vi "Other side RTS CTS Exchange.vi"() -> ()   [LabVIEW 2012]
uses:
  <instrlib>/niUSRP/niUSRP Fetch Rx Data (CDB).vi
  <vilib>/Analysis/2dsp.llb/Complex FFT.vi
  <vilib>/addons/Modulation/Digital/General/MT Map QAM Symbols to Bits.vi
  <vilib>/addons/Modulation/Digital/General/MT Map Bits to QAM Symbols.vi
  <instrlib>/niUSRP/niUSRP Write Tx Data (CDB).vi
  <vilib>/Analysis/2dsp.llb/Inverse Complex FFT.vi
  <vilib>/Waveform/DWDTOps.llb/DWDT Binary U8 to Digital.vi
  <vilib>/Waveform/DWDTOps.llb/DWDT Digital to Analog.vi
  <vilib>/Analysis/NI_AALPro.lvlib
  <vilib>/addons/Modulation/niDMT.lvlib
panel:
  out "Received Signal":waveform(dbl)(graph)
  out "analog waveform":waveform(dbl)
  out "CTS is send":bool
  out "sum":i8
  out "output array 2":i8[](array[numeric])
  out "output array 3":i8[](array[numeric])
  in  "stop":bool
  out "Reference Signal \n(RTS) Received":bool
  in  "Tab Control":enum32{"Parameters", "Debug", "CFO"}(tab)
  in  "Device names":refnum<k15>="192.168.10.3"
  in  "Active antenna":string="RX1"
  in  "Gain":dbl=3.0 format="%#_6f"
  in  "Carrier frequency":dbl=910000000.0 format="%#_6p"
  in  "IQ rate":dbl=5000000.0 format="%#_6p"
  in  "Number of samples":i64=1600
  out "Coerced IQ rate":dbl=100000.0 format="%#_6p"
  out "error out":errorcluster
  out "error out 2":errorcluster
  out "CFOest (Hz)":dbl[](array[numeric])
  out "Magnitude":dbl[](graph)
  out "Phase":dbl[](graph)
  out "FFT {X}":dbl[](graph)
  out "theta":dbl[](graph)
  out "Unequalized Data":cdb[](graph)
  out "Equalized Data":cdb[](graph)
  out "output bit stream":i8[][](array[numeric])
  out "Received Message":string
  out "millisecond timer to \n    Receive Signal":u32
  in  "Tab Control 2":enum32{"Parameters", "Debug"}(tab)
  out "coerced IQ rate":dbl=100000.0 format="%#_6p"
  in  "error in (no error)":errorcluster
  out "error out 3":errorcluster
  out "X":cdb[](array[numeric])
  out "Array out":cdb[](array[numeric])
  out "Interleaved Output":cdb[](array[numeric])
  out "Output with CP":cdb[](array[numeric])
  out "Data Size":i32
  out "Reference Symbols \n         Added":i32
  out "After Zero \n  Padding":i32
  out "After CP":i32
  out "Outgoing Constellation":cdb[](graph)=[-0.7071067811865476-0.7071067811865476i, -0.7071067811865476-0.7071067811865476i, -0.7071067811865476-0.7071067811865476i, 0.7071067811865476-0.7071067811865476i, 0.7071067811865476-0.7071067811865476i, 0.7071067811865476+0.7071067811865476i, 0.7071067811865476-0.7071067811865476i, -0.7071067811865476-0.7071067811865476i, 0.7071067811865476+0.7071067811865476i, -0.7071067811865476+0.7071067811865476i, -0.7071067811865476-0.7071067811865476i, -0.7071067811865476+0.7071067811865476i, -0.7071067811865476+0.7071067811865476i, 0.7071067811865476-0.7071067811865476i, -0.7071067811865476+0.7071067811865476i, -0.7071067811865476+0.7071067811865476i, 0.7071067811865476-0.7071067811865476i, -0.7071067811865476+0.7071067811865476i, -0.7071067811865476-0.7071067811865476i, 0.7071067811865476-0.7071067811865476i, 0.7071067811865476+0.7071067811865476i, -0.7071067811865476-0.7071067811865476i, -0.7071067811865476-0.7071067811865476i, 0.7071067811865476-0.7071067811865476i, -0.7071067811865476-0.7071067811865476i, 0.7071067811865476-0.7071067811865476i, 0.7071067811865476-0.7071067811865476i, 0.7071067811865476+0.7071067811865476i, 0.7071067811865476+0.7071067811865476i, -0.7071067811865476-0.7071067811865476i, -0.7071067811865476+0.7071067811865476i, -0.7071067811865476+0.7071067811865476i, 0.7071067811865476-0.7071067811865476i, -0.7071067811865476-0.7071067811865476i, -0.7071067811865476+0.7071067811865476i, -0.7071067811865476-0.7071067811865476i, -0.7071067811865476+0.7071067811865476i, 0.7071067811865476-0.7071067811865476i, 0.7071067811865476+0.7071067811865476i, 0.7071067811865476+0.7071067811865476i, 0.7071067811865476-0.7071067811865476i, -0.7071067811865476-0.7071067811865476i, -0.7071067811865476+0.7071067811865476i, -0.7071067811865476+0.7071067811865476i, -0.7071067811865476-0.7071067811865476i, -0.7071067811865476-0.7071067811865476i, -0.7071067811865476+0.7071067811865476i, -0.7071067811865476+0.7071067811865476i, -0.7071067811865476+0.7071067811865476i, -0.7071067811865476+0.7071067811865476i, 0.7071067811865476+0.7071067811865476i, 0.7071067811865476+0.7071067811865476i, 0.7071067811865476+0.7071067811865476i, 0.7071067811865476-0.7071067811865476i, 0.7071067811865476-0.7071067811865476i, -0.7071067811865476+0.7071067811865476i, -0.7071067811865476+0.7071067811865476i, -0.7071067811865476+0.7071067811865476i, -0.7071067811865476-0.7071067811865476i, 0.7071067811865476-0.7071067811865476i, -0.7071067811865476+0.7071067811865476i, -0.7071067811865476+0.7071067811865476i, -0.7071067811865476-0.7071067811865476i, -0.7071067811865476+0.7071067811865476i, -0.7071067811865476-0.7071067811865476i, 0.7071067811865476+0.7071067811865476i, 0.7071067811865476+0.7071067811865476i, 0.7071067811865476+0.7071067811865476i, -0.7071067811865476-0.7071067811865476i, 0.7071067811865476-0.7071067811865476i, -0.7071067811865476+0.7071067811865476i, -0.7071067811865476-0.7071067811865476i, -0.7071067811865476+0.7071067811865476i, 0.7071067811865476+0.7071067811865476i, 0.7071067811865476-0.7071067811865476i, -0.7071067811865476+0.7071067811865476i, -0.7071067811865476-0.7071067811865476i, 0.7071067811865476-0.7071067811865476i, 0.7071067811865476-0.7071067811865476i, -0.7071067811865476-0.7071067811865476i, 0.7071067811865476-0.7071067811865476i, 0.7071067811865476-0.7071067811865476i, 0.7071067811865476-0.7071067811865476i, 0.7071067811865476+0.7071067811865476i, 0.7071067811865476-0.7071067811865476i, -0.7071067811865476+0.7071067811865476i, 0.7071067811865476+0.7071067811865476i, 0.7071067811865476+0.7071067811865476i, -0.7071067811865476-0.7071067811865476i, 0.7071067811865476+0.7071067811865476i, -0.7071067811865476-0.7071067811865476i, 0.7071067811865476-0.7071067811865476i, 0.7071067811865476+0.7071067811865476i, -0.7071067811865476+0.7071067811865476i, -0.7071067811865476+0.7071067811865476i, -0.7071067811865476-0.7071067811865476i, 0.7071067811865476-0.7071067811865476i, -0.7071067811865476-0.7071067811865476i, -0.7071067811865476+0.7071067811865476i, 0.7071067811865476-0.7071067811865476i, -0.7071067811865476+0.7071067811865476i, 0.7071067811865476-0.7071067811865476i, 0.7071067811865476-0.7071067811865476i, 0.7071067811865476+0.7071067811865476i, -0.7071067811865476+0.7071067811865476i, -0.7071067811865476-0.7071067811865476i, -0.7071067811865476+0.7071067811865476i, -0.7071067811865476-0.7071067811865476i, 0.7071067811865476-0.7071067811865476i, 0.7071067811865476+0.7071067811865476i, -0.7071067811865476+0.7071067811865476i, -0.7071067811865476-0.7071067811865476i, -0.7071067811865476-0.7071067811865476i, -0.7071067811865476-0.7071067811865476i, -0.7071067811865476-0.7071067811865476i, 0.7071067811865476+0.7071067811865476i, 0.7071067811865476+0.7071067811865476i, -0.7071067811865476+0.7071067811865476i, -0.7071067811865476-0.7071067811865476i, 0.7071067811865476-0.7071067811865476i, -0.7071067811865476-0.7071067811865476i, -0.7071067811865476-0.7071067811865476i, 0.7071067811865476-0.7071067811865476i, 0.7071067811865476+0.7071067811865476i, 0.7071067811865476-0.7071067811865476i, -0.7071067811865476-0.7071067811865476i, 0.7071067811865476-0.7071067811865476i, -0.7071067811865476+0.7071067811865476i, 0.7071067811865476-0.7071067811865476i, -0.7071067811865476+0.7071067811865476i, 0.7071067811865476+0.7071067811865476i, 0.7071067811865476+0.7071067811865476i, -0.7071067811865476+0.7071067811865476i, 0.7071067811865476+0.7071067811865476i, 0.7071067811865476-0.7071067811865476i, 0.7071067811865476-0.7071067811865476i, -0.7071067811865476+0.7071067811865476i, -0.7071067811865476-0.7071067811865476i, -0.7071067811865476+0.7071067811865476i, 0.7071067811865476-0.7071067811865476i, 0.7071067811865476-0.7071067811865476i, 0.7071067811865476+0.7071067811865476i, -0.7071067811865476-0.7071067811865476i, -0.7071067811865476-0.7071067811865476i, 0.7071067811865476+0.7071067811865476i, -0.7071067811865476-0.7071067811865476i, -0.7071067811865476-0.7071067811865476i, 0.7071067811865476-0.7071067811865476i, -0.7071067811865476+0.7071067811865476i, 0.7071067811865476-0.7071067811865476i, -0.7071067811865476-0.7071067811865476i, 0.7071067811865476+0.7071067811865476i, -0.7071067811865476+0.7071067811865476i, -0.7071067811865476+0.7071067811865476i, -0.7071067811865476+0.7071067811865476i, 0.7071067811865476+0.7071067811865476i, 0.7071067811865476-0.7071067811865476i, 0.7071067811865476+0.7071067811865476i, -0.7071067811865476-0.7071067811865476i, 0.7071067811865476-0.7071067811865476i, 0.7071067811865476+0.7071067811865476i, -0.7071067811865476-0.7071067811865476i, -0.7071067811865476+0.7071067811865476i, 0.7071067811865476-0.7071067811865476i, 0.7071067811865476-0.7071067811865476i, 0.7071067811865476-0.7071067811865476i, -0.7071067811865476-0.7071067811865476i, 0.7071067811865476-0.7071067811865476i, 0.7071067811865476+0.7071067811865476i, 0.7071067811865476-0.7071067811865476i, -0.7071067811865476+0.7071067811865476i, 0.7071067811865476-0.7071067811865476i, 0.7071067811865476+0.7071067811865476i, 0.7071067811865476-0.7071067811865476i, 0.7071067811865476+0.7071067811865476i, 0.7071067811865476-0.7071067811865476i, 0.7071067811865476+0.7071067811865476i, 0.7071067811865476+0.7071067811865476i, 0.7071067811865476+0.7071067811865476i, -0.7071067811865476+0.7071067811865476i, 0.7071067811865476+0.7071067811865476i, 0.7071067811865476+0.7071067811865476i, 0.7071067811865476-0.7071067811865476i, 0.7071067811865476+0.7071067811865476i, -0.7071067811865476-0.7071067811865476i, 0.7071067811865476+0.7071067811865476i, 0.7071067811865476+0.7071067811865476i, 0.7071067811865476-0.7071067811865476i, -0.7071067811865476+0.7071067811865476i, -0.7071067811865476-0.7071067811865476i, 0.7071067811865476+0.7071067811865476i, 0.7071067811865476-0.7071067811865476i, 0.7071067811865476-0.7071067811865476i, 0.7071067811865476-0.7071067811865476i, -0.7071067811865476-0.7071067811865476i, 0.7071067811865476+0.7071067811865476i, 0.7071067811865476+0.7071067811865476i, -0.7071067811865476-0.7071067811865476i, -0.7071067811865476+0.7071067811865476i, -0.7071067811865476-0.7071067811865476i, 0.7071067811865476-0.7071067811865476i, 0.7071067811865476-0.7071067811865476i, -0.7071067811865476+0.7071067811865476i, 0.7071067811865476-0.7071067811865476i, -0.7071067811865476-0.7071067811865476i, 0.7071067811865476-0.7071067811865476i, -0.7071067811865476+0.7071067811865476i, 0.7071067811865476+0.7071067811865476i, -0.7071067811865476+0.7071067811865476i, -0.7071067811865476+0.7071067811865476i, 0.7071067811865476+0.7071067811865476i, 0.7071067811865476+0.7071067811865476i, 0.7071067811865476-0.7071067811865476i, 0.7071067811865476-0.7071067811865476i, -0.7071067811865476-0.7071067811865476i, -0.7071067811865476+0.7071067811865476i, 0.7071067811865476+0.7071067811865476i, -0.7071067811865476-0.7071067811865476i, -0.7071067811865476-0.7071067811865476i, -0.7071067811865476-0.7071067811865476i, -0.7071067811865476+0.7071067811865476i, 0.7071067811865476-0.7071067811865476i, -0.7071067811865476+0.7071067811865476i, 0.7071067811865476+0.7071067811865476i, 0.7071067811865476-0.7071067811865476i, -0.7071067811865476+0.7071067811865476i, -0.7071067811865476+0.7071067811865476i, 0.7071067811865476-0.7071067811865476i, -0.7071067811865476-0.7071067811865476i, -0.7071067811865476-0.7071067811865476i, -0.7071067811865476-0.7071067811865476i, 0.7071067811865476+0.7071067811865476i, 0.7071067811865476-0.7071067811865476i, -0.7071067811865476+0.7071067811865476i, 0.7071067811865476-0.7071067811865476i, 0.7071067811865476-0.7071067811865476i, 0.7071067811865476-0.7071067811865476i, -0.7071067811865476+0.7071067811865476i, 0.7071067811865476-0.7071067811865476i, -0.7071067811865476+0.7071067811865476i, 0.7071067811865476-0.7071067811865476i, 0.7071067811865476+0.7071067811865476i, 0.7071067811865476+0.7071067811865476i, 0.7071067811865476+0.7071067811865476i, -0.7071067811865476-0.7071067811865476i, 0.7071067811865476+0.7071067811865476i, -0.7071067811865476+0.7071067811865476i, 0.7071067811865476-0.7071067811865476i, -0.7071067811865476+0.7071067811865476i, -0.7071067811865476+0.7071067811865476i, 0.7071067811865476+0.7071067811865476i, -0.7071067811865476+0.7071067811865476i, 0.7071067811865476-0.7071067811865476i, 0.7071067811865476-0.7071067811865476i, -0.7071067811865476+0.7071067811865476i, -0.7071067811865476+0.7071067811865476i, -0.7071067811865476-0.7071067811865476i, -0.7071067811865476-0.7071067811865476i, -0.7071067811865476-0.7071067811865476i, -0.7071067811865476+0.7071067811865476i, 0.7071067811865476+0.7071067811865476i, -0.7071067811865476+0.7071067811865476i, -0.7071067811865476+0.7071067811865476i, 0.7071067811865476-0.7071067811865476i, 0.7071067811865476+0.7071067811865476i, -0.7071067811865476-0.7071067811865476i, 0.7071067811865476-0.7071067811865476i, 0.7071067811865476-0.7071067811865476i, -0.7071067811865476-0.7071067811865476i, 0.7071067811865476+0.7071067811865476i, 0.7071067811865476-0.7071067811865476i, -0.7071067811865476-0.7071067811865476i, 0.7071067811865476+0.7071067811865476i, -0.7071067811865476-0.7071067811865476i, -0.7071067811865476-0.7071067811865476i, 0.7071067811865476+0.7071067811865476i, -0.7071067811865476+0.7071067811865476i, -0.7071067811865476-0.7071067811865476i, -0.7071067811865476-0.7071067811865476i, -0.7071067811865476+0.7071067811865476i, -0.7071067811865476-0.7071067811865476i, -0.7071067811865476+0.7071067811865476i, 0.7071067811865476+0.7071067811865476i, 0.7071067811865476+0.7071067811865476i, -0.7071067811865476+0.7071067811865476i, 0.7071067811865476-0.7071067811865476i, 0.7071067811865476-0.7071067811865476i, -0.7071067811865476-0.7071067811865476i, -0.7071067811865476+0.7071067811865476i, 0.7071067811865476-0.7071067811865476i, -0.7071067811865476-0.7071067811865476i, 0.7071067811865476-0.7071067811865476i, -0.7071067811865476-0.7071067811865476i, 0.7071067811865476+0.7071067811865476i, 0.7071067811865476+0.7071067811865476i, -0.7071067811865476+0.7071067811865476i, -0.7071067811865476+0.7071067811865476i, 0.7071067811865476-0.7071067811865476i, 0.7071067811865476-0.7071067811865476i, -0.7071067811865476-0.7071067811865476i, -0.7071067811865476-0.7071067811865476i, 0.7071067811865476-0.7071067811865476i, 0.7071067811865476-0.7071067811865476i, 0.7071067811865476-0.7071067811865476i, 0.7071067811865476-0.7071067811865476i, 0.7071067811865476-0.7071067811865476i, 0.7071067811865476+0.7071067811865476i, 0.7071067811865476+0.7071067811865476i, -0.7071067811865476+0.7071067811865476i, -0.7071067811865476+0.7071067811865476i, 0.7071067811865476+0.7071067811865476i, 0.7071067811865476-0.7071067811865476i, 0.7071067811865476-0.7071067811865476i, -0.7071067811865476-0.7071067811865476i, -0.7071067811865476-0.7071067811865476i, 0.7071067811865476+0.7071067811865476i, 0.7071067811865476-0.7071067811865476i, -0.7071067811865476-0.7071067811865476i, 0.7071067811865476-0.7071067811865476i, -0.7071067811865476-0.7071067811865476i, 0.7071067811865476-0.7071067811865476i, 0.7071067811865476+0.7071067811865476i, 0.7071067811865476+0.7071067811865476i, -0.7071067811865476+0.7071067811865476i, -0.7071067811865476-0.7071067811865476i, 0.7071067811865476+0.7071067811865476i, -0.7071067811865476-0.7071067811865476i, 0.7071067811865476-0.7071067811865476i, 0.7071067811865476-0.7071067811865476i, -0.7071067811865476+0.7071067811865476i, 0.7071067811865476+0.7071067811865476i, -0.7071067811865476-0.7071067811865476i, -0.7071067811865476-0.7071067811865476i, -0.7071067811865476+0.7071067811865476i, -0.7071067811865476+0.7071067811865476i, -0.7071067811865476-0.7071067811865476i, -0.7071067811865476+0.7071067811865476i, -0.7071067811865476+0.7071067811865476i, 0.7071067811865476+0.7071067811865476i, -0.7071067811865476+0.7071067811865476i, 0.7071067811865476+0.7071067811865476i, 0.7071067811865476-0.7071067811865476i, 0.7071067811865476+0.7071067811865476i, -0.7071067811865476+0.7071067811865476i, 0.7071067811865476-0.7071067811865476i, -0.7071067811865476+0.7071067811865476i, -0.7071067811865476-0.7071067811865476i, 0.7071067811865476+0.7071067811865476i, 0.7071067811865476+0.7071067811865476i, 0.7071067811865476-0.7071067811865476i, -0.7071067811865476-0.7071067811865476i, -0.7071067811865476-0.7071067811865476i, -0.7071067811865476+0.7071067811865476i, 0.7071067811865476-0.7071067811865476i, -0.7071067811865476-0.7071067811865476i, 0.7071067811865476+0.7071067811865476i, -0.7071067811865476-0.7071067811865476i, -0.7071067811865476+0.7071067811865476i, 0.7071067811865476+0.7071067811865476i, 0.7071067811865476+0.7071067811865476i, -0.7071067811865476-0.7071067811865476i, 0.7071067811865476-0.7071067811865476i, -0.7071067811865476-0.7071067811865476i, -0.7071067811865476-0.7071067811865476i, 0.7071067811865476+0.7071067811865476i, 0.7071067811865476+0.7071067811865476i, -0.7071067811865476-0.7071067811865476i, -0.7071067811865476-0.7071067811865476i, -0.7071067811865476-0.7071067811865476i, -0.7071067811865476-0.7071067811865476i, 0.7071067811865476-0.7071067811865476i, 0.7071067811865476+0.7071067811865476i, 0.7071067811865476+0.7071067811865476i, -0.7071067811865476-0.7071067811865476i, -0.7071067811865476-0.7071067811865476i, -0.7071067811865476+0.7071067811865476i, -0.7071067811865476-0.7071067811865476i, -0.7071067811865476-0.7071067811865476i, 0.7071067811865476+0.7071067811865476i, -0.7071067811865476+0.7071067811865476i, -0.7071067811865476+0.7071067811865476i, -0.7071067811865476-0.7071067811865476i, 0.7071067811865476+0.7071067811865476i, -0.7071067811865476-0.7071067811865476i, 0.7071067811865476+0.7071067811865476i, 0.7071067811865476-0.7071067811865476i, 0.7071067811865476+0.7071067811865476i, 0.7071067811865476+0.7071067811865476i, 0.7071067811865476-0.7071067811865476i, -0.7071067811865476+0.7071067811865476i, -0.7071067811865476+0.7071067811865476i, 0.7071067811865476+0.7071067811865476i, -0.7071067811865476-0.7071067811865476i, 0.7071067811865476-0.7071067811865476i, -0.7071067811865476-0.7071067811865476i, -0.7071067811865476+0.7071067811865476i, 0.7071067811865476+0.7071067811865476i, -0.7071067811865476+0.7071067811865476i, -0.7071067811865476-0.7071067811865476i, 0.7071067811865476-0.7071067811865476i, -0.7071067811865476+0.7071067811865476i, -0.7071067811865476-0.7071067811865476i, -0.7071067811865476-0.7071067811865476i, 0.7071067811865476+0.7071067811865476i, -0.7071067811865476-0.7071067811865476i, -0.7071067811865476+0.7071067811865476i, 0.7071067811865476-0.7071067811865476i, 0.7071067811865476+0.7071067811865476i, 0.7071067811865476-0.7071067811865476i, 0.7071067811865476-0.7071067811865476i, 0.7071067811865476-0.7071067811865476i, -0.7071067811865476+0.7071067811865476i, 0.7071067811865476+0.7071067811865476i, -0.7071067811865476+0.7071067811865476i, -0.7071067811865476-0.7071067811865476i, 0.7071067811865476+0.7071067811865476i, -0.7071067811865476+0.7071067811865476i, 0.7071067811865476-0.7071067811865476i, -0.7071067811865476-0.7071067811865476i, -0.7071067811865476+0.7071067811865476i, -0.7071067811865476+0.7071067811865476i, -0.7071067811865476+0.7071067811865476i, -0.7071067811865476-0.7071067811865476i, 0.7071067811865476+0.7071067811865476i, -0.7071067811865476+0.7071067811865476i, 0.7071067811865476+0.7071067811865476i, -0.7071067811865476-0.7071067811865476i, 0.7071067811865476+0.7071067811865476i, -0.7071067811865476+0.7071067811865476i, 0.7071067811865476+0.7071067811865476i, -0.7071067811865476+0.7071067811865476i, 0.7071067811865476+0.7071067811865476i, 0.7071067811865476+0.7071067811865476i, 0.7071067811865476+0.7071067811865476i, 0.7071067811865476+0.7071067811865476i, 0.7071067811865476-0.7071067811865476i, 0.7071067811865476+0.7071067811865476i, -0.7071067811865476+0.7071067811865476i, 0.7071067811865476+0.7071067811865476i, -0.7071067811865476+0.7071067811865476i, 0.7071067811865476-0.7071067811865476i, 0.7071067811865476+0.7071067811865476i, -0.7071067811865476+0.7071067811865476i, 0.7071067811865476+0.7071067811865476i, -0.7071067811865476-0.7071067811865476i, 0.7071067811865476-0.7071067811865476i, -0.7071067811865476+0.7071067811865476i, -0.7071067811865476+0.7071067811865476i, -0.7071067811865476+0.7071067811865476i, -0.7071067811865476+0.7071067811865476i, 0.7071067811865476-0.7071067811865476i, 0.7071067811865476+0.7071067811865476i, -0.7071067811865476+0.7071067811865476i, 0.7071067811865476-0.7071067811865476i, -0.7071067811865476-0.7071067811865476i, -0.7071067811865476-0.7071067811865476i, -0.7071067811865476+0.7071067811865476i, 0.7071067811865476+0.7071067811865476i, -0.7071067811865476-0.7071067811865476i, -0.7071067811865476+0.7071067811865476i, -0.7071067811865476-0.7071067811865476i, 0.7071067811865476+0.7071067811865476i, 0.7071067811865476-0.7071067811865476i, 0.7071067811865476+0.7071067811865476i, 0.7071067811865476-0.7071067811865476i, 0.7071067811865476-0.7071067811865476i, 0.7071067811865476+0.7071067811865476i, -0.7071067811865476+0.7071067811865476i, -0.7071067811865476+0.7071067811865476i, -0.7071067811865476+0.7071067811865476i, 0.7071067811865476-0.7071067811865476i, 0.7071067811865476-0.7071067811865476i, -0.7071067811865476+0.7071067811865476i, -0.7071067811865476-0.7071067811865476i, -0.7071067811865476-0.7071067811865476i, 0.7071067811865476-0.7071067811865476i, -0.7071067811865476-0.7071067811865476i, 0.7071067811865476+0.7071067811865476i, 0.7071067811865476-0.7071067811865476i, -0.7071067811865476+0.7071067811865476i, 0.7071067811865476+0.7071067811865476i, 0.7071067811865476-0.7071067811865476i, -0.7071067811865476-0.7071067811865476i, -0.7071067811865476+0.7071067811865476i, -0.7071067811865476-0.7071067811865476i, -0.7071067811865476-0.7071067811865476i, 0.7071067811865476-0.7071067811865476i, -0.7071067811865476+0.7071067811865476i, 0.7071067811865476+0.7071067811865476i, -0.7071067811865476-0.7071067811865476i, -0.7071067811865476+0.7071067811865476i, -0.7071067811865476+0.7071067811865476i, 0.7071067811865476+0.7071067811865476i, -0.7071067811865476-0.7071067811865476i, 0.7071067811865476+0.7071067811865476i, -0.7071067811865476-0.7071067811865476i, 0.7071067811865476+0.7071067811865476i, 0.7071067811865476+0.7071067811865476i, 0.7071067811865476+0.7071067811865476i, -0.7071067811865476+0.7071067811865476i, 0.7071067811865476-0.7071067811865476i, 0.7071067811865476+0.7071067811865476i, -0.7071067811865476-0.7071067811865476i, 0.7071067811865476+0.7071067811865476i, 0.7071067811865476-0.7071067811865476i, 0.7071067811865476-0.7071067811865476i, 0.7071067811865476+0.7071067811865476i, -0.7071067811865476-0.7071067811865476i, -0.7071067811865476+0.7071067811865476i, 0.7071067811865476+0.7071067811865476i, 0.7071067811865476-0.7071067811865476i, -0.7071067811865476-0.7071067811865476i, -0.7071067811865476-0.7071067811865476i, -0.7071067811865476-0.7071067811865476i, 0.7071067811865476-0.7071067811865476i, 0.7071067811865476-0.7071067811865476i, 0.7071067811865476+0.7071067811865476i, 0.7071067811865476-0.7071067811865476i, -0.7071067811865476-0.7071067811865476i, 0.7071067811865476+0.7071067811865476i, -0.7071067811865476+0.7071067811865476i, -0.7071067811865476-0.7071067811865476i, -0.7071067811865476+0.7071067811865476i, -0.7071067811865476+0.7071067811865476i, 0.7071067811865476-0.7071067811865476i, -0.7071067811865476+0.7071067811865476i, -0.7071067811865476+0.7071067811865476i, 0.7071067811865476-0.7071067811865476i, -0.7071067811865476+0.7071067811865476i, -0.7071067811865476-0.7071067811865476i, 0.7071067811865476-0.7071067811865476i, 0.7071067811865476+0.7071067811865476i, -0.7071067811865476-0.7071067811865476i, -0.7071067811865476-0.7071067811865476i, 0.7071067811865476-0.7071067811865476i, -0.7071067811865476-0.7071067811865476i, 0.7071067811865476-0.7071067811865476i, 0.7071067811865476-0.7071067811865476i, 0.7071067811865476+0.7071067811865476i, 0.7071067811865476+0.7071067811865476i, -0.7071067811865476-0.7071067811865476i, -0.7071067811865476+0.7071067811865476i, -0.7071067811865476+0.7071067811865476i, 0.7071067811865476-0.7071067811865476i, -0.7071067811865476-0.7071067811865476i, -0.7071067811865476+0.7071067811865476i, -0.7071067811865476-0.7071067811865476i, -0.7071067811865476+0.7071067811865476i, 0.7071067811865476-0.7071067811865476i, 0.7071067811865476+0.7071067811865476i, 0.7071067811865476+0.7071067811865476i, 0.7071067811865476-0.7071067811865476i, -0.7071067811865476-0.7071067811865476i, -0.7071067811865476+0.7071067811865476i, -0.7071067811865476+0.7071067811865476i, -0.7071067811865476-0.7071067811865476i, -0.7071067811865476-0.7071067811865476i, -0.7071067811865476+0.7071067811865476i, -0.7071067811865476+0.7071067811865476i, -0.7071067811865476+0.7071067811865476i, -0.7071067811865476+0.7071067811865476i, 0.7071067811865476+0.7071067811865476i, 0.7071067811865476+0.7071067811865476i, 0.7071067811865476+0.7071067811865476i, 0.7071067811865476-0.7071067811865476i, 0.7071067811865476-0.7071067811865476i, -0.7071067811865476+0.7071067811865476i, -0.7071067811865476+0.7071067811865476i, -0.7071067811865476+0.7071067811865476i, -0.7071067811865476-0.7071067811865476i, 0.7071067811865476-0.7071067811865476i, -0.7071067811865476+0.7071067811865476i, -0.7071067811865476+0.7071067811865476i, -0.7071067811865476-0.7071067811865476i, -0.7071067811865476+0.7071067811865476i, -0.7071067811865476-0.7071067811865476i, 0.7071067811865476+0.7071067811865476i, 0.7071067811865476+0.7071067811865476i, 0.7071067811865476+0.7071067811865476i, -0.7071067811865476-0.7071067811865476i, 0.7071067811865476-0.7071067811865476i, -0.7071067811865476+0.7071067811865476i, -0.7071067811865476-0.7071067811865476i, -0.7071067811865476+0.7071067811865476i, 0.7071067811865476+0.7071067811865476i, 0.7071067811865476-0.7071067811865476i, -0.7071067811865476+0.7071067811865476i, -0.7071067811865476-0.7071067811865476i, 0.7071067811865476-0.7071067811865476i, 0.7071067811865476-0.7071067811865476i, -0.7071067811865476-0.7071067811865476i, 0.7071067811865476-0.7071067811865476i, 0.7071067811865476-0.7071067811865476i, 0.7071067811865476-0.7071067811865476i, 0.7071067811865476+0.7071067811865476i, 0.7071067811865476-0.7071067811865476i, -0.7071067811865476+0.7071067811865476i, 0.7071067811865476+0.7071067811865476i, 0.7071067811865476+0.7071067811865476i, -0.7071067811865476-0.7071067811865476i, 0.7071067811865476+0.7071067811865476i, -0.7071067811865476-0.7071067811865476i, 0.7071067811865476-0.7071067811865476i, 0.7071067811865476+0.7071067811865476i, -0.7071067811865476+0.7071067811865476i, -0.7071067811865476+0.7071067811865476i, -0.7071067811865476-0.7071067811865476i, 0.7071067811865476-0.7071067811865476i, -0.7071067811865476-0.7071067811865476i, -0.7071067811865476+0.7071067811865476i, 0.7071067811865476-0.7071067811865476i, -0.7071067811865476+0.7071067811865476i, 0.7071067811865476-0.7071067811865476i, 0.7071067811865476-0.7071067811865476i, 0.7071067811865476+0.7071067811865476i, -0.7071067811865476+0.7071067811865476i, -0.7071067811865476-0.7071067811865476i, -0.7071067811865476+0.7071067811865476i, -0.7071067811865476-0.7071067811865476i, 0.7071067811865476-0.7071067811865476i, 0.7071067811865476+0.7071067811865476i, -0.7071067811865476+0.7071067811865476i, -0.7071067811865476-0.7071067811865476i, -0.7071067811865476-0.7071067811865476i, -0.7071067811865476-0.7071067811865476i, -0.7071067811865476-0.7071067811865476i, 0.7071067811865476+0.7071067811865476i, 0.7071067811865476+0.7071067811865476i, -0.7071067811865476+0.7071067811865476i, -0.7071067811865476-0.7071067811865476i, 0.7071067811865476-0.7071067811865476i, -0.7071067811865476-0.7071067811865476i, -0.7071067811865476-0.7071067811865476i, 0.7071067811865476-0.7071067811865476i, 0.7071067811865476+0.7071067811865476i, 0.7071067811865476-0.7071067811865476i, -0.7071067811865476-0.7071067811865476i, 0.7071067811865476-0.7071067811865476i, -0.7071067811865476+0.7071067811865476i, 0.7071067811865476-0.7071067811865476i, -0.7071067811865476+0.7071067811865476i, 0.7071067811865476+0.7071067811865476i, 0.7071067811865476+0.7071067811865476i, -0.7071067811865476+0.7071067811865476i, 0.7071067811865476+0.7071067811865476i, 0.7071067811865476-0.7071067811865476i, 0.7071067811865476-0.7071067811865476i, -0.7071067811865476+0.7071067811865476i, -0.7071067811865476-0.7071067811865476i, -0.7071067811865476+0.7071067811865476i, 0.7071067811865476-0.7071067811865476i, 0.7071067811865476-0.7071067811865476i, 0.7071067811865476+0.7071067811865476i, -0.7071067811865476-0.7071067811865476i, -0.7071067811865476-0.7071067811865476i, 0.7071067811865476+0.7071067811865476i, -0.7071067811865476-0.7071067811865476i, -0.7071067811865476-0.7071067811865476i, 0.7071067811865476-0.7071067811865476i, -0.7071067811865476+0.7071067811865476i, 0.7071067811865476-0.7071067811865476i, -0.7071067811865476-0.7071067811865476i, 0.7071067811865476+0.7071067811865476i, -0.7071067811865476+0.7071067811865476i, -0.7071067811865476+0.7071067811865476i, -0.7071067811865476+0.7071067811865476i, 0.7071067811865476+0.7071067811865476i, 0.7071067811865476-0.7071067811865476i, 0.7071067811865476+0.7071067811865476i, -0.7071067811865476-0.7071067811865476i, 0.7071067811865476-0.7071067811865476i, 0.7071067811865476+0.7071067811865476i, -0.7071067811865476-0.7071067811865476i, -0.7071067811865476+0.7071067811865476i, 0.7071067811865476-0.7071067811865476i, 0.7071067811865476-0.7071067811865476i, 0.7071067811865476-0.7071067811865476i, -0.7071067811865476-0.7071067811865476i, 0.7071067811865476-0.7071067811865476i, 0.7071067811865476+0.7071067811865476i, 0.7071067811865476-0.7071067811865476i, -0.7071067811865476+0.7071067811865476i, 0.7071067811865476-0.7071067811865476i, 0.7071067811865476+0.7071067811865476i, 0.7071067811865476-0.7071067811865476i, 0.7071067811865476+0.7071067811865476i, 0.7071067811865476-0.7071067811865476i, 0.7071067811865476+0.7071067811865476i, 0.7071067811865476+0.7071067811865476i, 0.7071067811865476+0.7071067811865476i, -0.7071067811865476+0.7071067811865476i, 0.7071067811865476+0.7071067811865476i, 0.7071067811865476+0.7071067811865476i, 0.7071067811865476-0.7071067811865476i, 0.7071067811865476+0.7071067811865476i, -0.7071067811865476-0.7071067811865476i, 0.7071067811865476+0.7071067811865476i, 0.7071067811865476+0.7071067811865476i, 0.7071067811865476-0.7071067811865476i, -0.7071067811865476+0.7071067811865476i, -0.7071067811865476-0.7071067811865476i, 0.7071067811865476+0.7071067811865476i, 0.7071067811865476-0.7071067811865476i, 0.7071067811865476-0.7071067811865476i, 0.7071067811865476-0.7071067811865476i, -0.7071067811865476-0.7071067811865476i, 0.7071067811865476+0.7071067811865476i, 0.7071067811865476+0.7071067811865476i, -0.7071067811865476-0.7071067811865476i, -0.7071067811865476+0.7071067811865476i, -0.7071067811865476-0.7071067811865476i, 0.7071067811865476-0.7071067811865476i, 0.7071067811865476-0.7071067811865476i, -0.7071067811865476+0.7071067811865476i, 0.7071067811865476-0.7071067811865476i, -0.7071067811865476-0.7071067811865476i, 0.7071067811865476-0.7071067811865476i, -0.7071067811865476+0.7071067811865476i, 0.7071067811865476+0.7071067811865476i, -0.7071067811865476+0.7071067811865476i, -0.7071067811865476+0.7071067811865476i, 0.7071067811865476+0.7071067811865476i, 0.7071067811865476+0.7071067811865476i, 0.7071067811865476-0.7071067811865476i, 0.7071067811865476-0.7071067811865476i, -0.7071067811865476-0.7071067811865476i, -0.7071067811865476+0.7071067811865476i, 0.7071067811865476+0.7071067811865476i, -0.7071067811865476-0.7071067811865476i, -0.7071067811865476-0.7071067811865476i, -0.7071067811865476-0.7071067811865476i, -0.7071067811865476+0.7071067811865476i, 0.7071067811865476-0.7071067811865476i, -0.7071067811865476+0.7071067811865476i, 0.7071067811865476+0.7071067811865476i, 0.7071067811865476-0.7071067811865476i, -0.7071067811865476+0.7071067811865476i, -0.7071067811865476+0.7071067811865476i, 0.7071067811865476-0.7071067811865476i, -0.7071067811865476-0.7071067811865476i, -0.7071067811865476-0.7071067811865476i, -0.7071067811865476-0.7071067811865476i, 0.7071067811865476+0.7071067811865476i, 0.7071067811865476-0.7071067811865476i, -0.7071067811865476+0.7071067811865476i, 0.7071067811865476-0.7071067811865476i, 0.7071067811865476-0.7071067811865476i, 0.7071067811865476-0.7071067811865476i, -0.7071067811865476+0.7071067811865476i, 0.7071067811865476-0.7071067811865476i, -0.7071067811865476+0.7071067811865476i, 0.7071067811865476-0.7071067811865476i, 0.7071067811865476+0.7071067811865476i, 0.7071067811865476+0.7071067811865476i, 0.7071067811865476+0.7071067811865476i, -0.7071067811865476-0.7071067811865476i, 0.7071067811865476+0.7071067811865476i, -0.7071067811865476+0.7071067811865476i, 0.7071067811865476-0.7071067811865476i, -0.7071067811865476+0.7071067811865476i, -0.7071067811865476+0.7071067811865476i, 0.7071067811865476+0.7071067811865476i, -0.7071067811865476+0.7071067811865476i, 0.7071067811865476-0.7071067811865476i, 0.7071067811865476-0.7071067811865476i, -0.7071067811865476+0.7071067811865476i, -0.7071067811865476+0.7071067811865476i, -0.7071067811865476-0.7071067811865476i, -0.7071067811865476-0.7071067811865476i, -0.7071067811865476-0.7071067811865476i, -0.7071067811865476+0.7071067811865476i, 0.7071067811865476+0.7071067811865476i, -0.7071067811865476+0.7071067811865476i, -0.7071067811865476+0.7071067811865476i, 0.7071067811865476-0.7071067811865476i, 0.7071067811865476+0.7071067811865476i, -0.7071067811865476-0.7071067811865476i, 0.7071067811865476-0.7071067811865476i, 0.7071067811865476-0.7071067811865476i, -0.7071067811865476-0.7071067811865476i, 0.7071067811865476+0.7071067811865476i, 0.7071067811865476-0.7071067811865476i, -0.7071067811865476-0.7071067811865476i, 0.7071067811865476+0.7071067811865476i, -0.7071067811865476-0.7071067811865476i, -0.7071067811865476-0.7071067811865476i, 0.7071067811865476+0.7071067811865476i, -0.7071067811865476+0.7071067811865476i, -0.7071067811865476-0.7071067811865476i, -0.7071067811865476-0.7071067811865476i, -0.7071067811865476+0.7071067811865476i, -0.7071067811865476-0.7071067811865476i, -0.7071067811865476+0.7071067811865476i, 0.7071067811865476+0.7071067811865476i, 0.7071067811865476+0.7071067811865476i, -0.7071067811865476+0.7071067811865476i, 0.7071067811865476-0.7071067811865476i, 0.7071067811865476-0.7071067811865476i, -0.7071067811865476-0.7071067811865476i, -0.7071067811865476+0.7071067811865476i, 0.7071067811865476-0.7071067811865476i, -0.7071067811865476-0.7071067811865476i, 0.7071067811865476-0.7071067811865476i, -0.7071067811865476-0.7071067811865476i, 0.7071067811865476+0.7071067811865476i, 0.7071067811865476+0.7071067811865476i, -0.7071067811865476+0.7071067811865476i, -0.7071067811865476+0.7071067811865476i, 0.7071067811865476-0.7071067811865476i, 0.7071067811865476-0.7071067811865476i, -0.7071067811865476-0.7071067811865476i, -0.7071067811865476-0.7071067811865476i, 0.7071067811865476-0.7071067811865476i, 0.7071067811865476-0.7071067811865476i, 0.7071067811865476-0.7071067811865476i, 0.7071067811865476-0.7071067811865476i, 0.7071067811865476-0.7071067811865476i, 0.7071067811865476+0.7071067811865476i, 0.7071067811865476+0.7071067811865476i, -0.7071067811865476+0.7071067811865476i, -0.7071067811865476+0.7071067811865476i, 0.7071067811865476+0.7071067811865476i, 0.7071067811865476-0.7071067811865476i, 0.7071067811865476-0.7071067811865476i, -0.7071067811865476-0.7071067811865476i, -0.7071067811865476-0.7071067811865476i, 0.7071067811865476+0.7071067811865476i, 0.7071067811865476-0.7071067811865476i, -0.7071067811865476-0.7071067811865476i, 0.7071067811865476-0.7071067811865476i, -0.7071067811865476-0.7071067811865476i, 0.7071067811865476-0.7071067811865476i, 0.7071067811865476+0.7071067811865476i, 0.7071067811865476+0.7071067811865476i, -0.7071067811865476+0.7071067811865476i, -0.7071067811865476-0.7071067811865476i, 0.7071067811865476+0.7071067811865476i, -0.7071067811865476-0.7071067811865476i, 0.7071067811865476-0.7071067811865476i, 0.7071067811865476-0.7071067811865476i, -0.7071067811865476+0.7071067811865476i, 0.7071067811865476+0.7071067811865476i, -0.7071067811865476-0.7071067811865476i, -0.7071067811865476-0.7071067811865476i, -0.7071067811865476+0.7071067811865476i, -0.7071067811865476+0.7071067811865476i, -0.7071067811865476-0.7071067811865476i, -0.7071067811865476+0.7071067811865476i, -0.7071067811865476+0.7071067811865476i, 0.7071067811865476+0.7071067811865476i, -0.7071067811865476+0.7071067811865476i, 0.7071067811865476+0.7071067811865476i, 0.7071067811865476-0.7071067811865476i, 0.7071067811865476+0.7071067811865476i, -0.7071067811865476+0.7071067811865476i, 0.7071067811865476-0.7071067811865476i, -0.7071067811865476+0.7071067811865476i, -0.7071067811865476-0.7071067811865476i, 0.7071067811865476+0.7071067811865476i, 0.7071067811865476+0.7071067811865476i, 0.7071067811865476-0.7071067811865476i, -0.7071067811865476-0.7071067811865476i, -0.7071067811865476-0.7071067811865476i, -0.7071067811865476+0.7071067811865476i, 0.7071067811865476-0.7071067811865476i, -0.7071067811865476-0.7071067811865476i, 0.7071067811865476+0.7071067811865476i, -0.7071067811865476-0.7071067811865476i, -0.7071067811865476+0.7071067811865476i, 0.7071067811865476+0.7071067811865476i, 0.7071067811865476+0.7071067811865476i, -0.7071067811865476-0.7071067811865476i, 0.7071067811865476-0.7071067811865476i, -0.7071067811865476-0.7071067811865476i, -0.7071067811865476-0.7071067811865476i, 0.7071067811865476+0.7071067811865476i, 0.7071067811865476+0.7071067811865476i, -0.7071067811865476-0.7071067811865476i, -0.7071067811865476-0.7071067811865476i, -0.7071067811865476-0.7071067811865476i, -0.7071067811865476-0.7071067811865476i, 0.7071067811865476-0.7071067811865476i, 0.7071067811865476+0.7071067811865476i, 0.7071067811865476+0.7071067811865476i, -0.7071067811865476-0.7071067811865476i, -0.7071067811865476-0.7071067811865476i, -0.7071067811865476+0.7071067811865476i, -0.7071067811865476-0.7071067811865476i, -0.7071067811865476-0.7071067811865476i, 0.7071067811865476+0.7071067811865476i, -0.7071067811865476+0.7071067811865476i, -0.7071067811865476+0.7071067811865476i, -0.7071067811865476-0.7071067811865476i, 0.7071067811865476+0.7071067811865476i, -0.7071067811865476-0.7071067811865476i, 0.7071067811865476+0.7071067811865476i, 0.7071067811865476-0.7071067811865476i, 0.7071067811865476+0.7071067811865476i, 0.7071067811865476+0.7071067811865476i, 0.7071067811865476-0.7071067811865476i, -0.7071067811865476+0.7071067811865476i, -0.7071067811865476+0.7071067811865476i, 0.7071067811865476+0.7071067811865476i, -0.7071067811865476-0.7071067811865476i, 0.7071067811865476-0.7071067811865476i, -0.7071067811865476-0.7071067811865476i, -0.7071067811865476+0.7071067811865476i, 0.7071067811865476+0.7071067811865476i, -0.7071067811865476+0.7071067811865476i, -0.7071067811865476-0.7071067811865476i, 0.7071067811865476-0.7071067811865476i, -0.7071067811865476+0.7071067811865476i, -0.7071067811865476-0.7071067811865476i, -0.7071067811865476-0.7071067811865476i, 0.7071067811865476+0.7071067811865476i, -0.7071067811865476-0.7071067811865476i, -0.7071067811865476+0.7071067811865476i, 0.7071067811865476-0.7071067811865476i, 0.7071067811865476+0.7071067811865476i, 0.7071067811865476-0.7071067811865476i, 0.7071067811865476-0.7071067811865476i, 0.7071067811865476-0.7071067811865476i, -0.7071067811865476+0.7071067811865476i, 0.7071067811865476+0.7071067811865476i, -0.7071067811865476+0.7071067811865476i, -0.7071067811865476-0.7071067811865476i, 0.7071067811865476+0.7071067811865476i, -0.7071067811865476+0.7071067811865476i, 0.7071067811865476-0.7071067811865476i, -0.7071067811865476-0.7071067811865476i, -0.7071067811865476+0.7071067811865476i, -0.7071067811865476+0.7071067811865476i, -0.7071067811865476+0.7071067811865476i, -0.7071067811865476-0.7071067811865476i, 0.7071067811865476+0.7071067811865476i, -0.7071067811865476+0.7071067811865476i, 0.7071067811865476+0.7071067811865476i, -0.7071067811865476-0.7071067811865476i, 0.7071067811865476+0.7071067811865476i, -0.7071067811865476+0.7071067811865476i, 0.7071067811865476+0.7071067811865476i, -0.7071067811865476+0.7071067811865476i, 0.7071067811865476+0.7071067811865476i, 0.7071067811865476+0.7071067811865476i, 0.7071067811865476+0.7071067811865476i, 0.7071067811865476+0.7071067811865476i, 0.7071067811865476-0.7071067811865476i, 0.7071067811865476+0.7071067811865476i, -0.7071067811865476+0.7071067811865476i, 0.7071067811865476+0.7071067811865476i, -0.7071067811865476+0.7071067811865476i, 0.7071067811865476-0.7071067811865476i, 0.7071067811865476+0.7071067811865476i, -0.7071067811865476+0.7071067811865476i, 0.7071067811865476+0.7071067811865476i, -0.7071067811865476-0.7071067811865476i, 0.7071067811865476-0.7071067811865476i, -0.7071067811865476+0.7071067811865476i, -0.7071067811865476+0.7071067811865476i, -0.7071067811865476+0.7071067811865476i, -0.7071067811865476+0.7071067811865476i, 0.7071067811865476-0.7071067811865476i, 0.7071067811865476+0.7071067811865476i, -0.7071067811865476+0.7071067811865476i, 0.7071067811865476-0.7071067811865476i, -0.7071067811865476-0.7071067811865476i, -0.7071067811865476-0.7071067811865476i, -0.7071067811865476+0.7071067811865476i, 0.7071067811865476+0.7071067811865476i, -0.7071067811865476-0.7071067811865476i, -0.7071067811865476+0.7071067811865476i, -0.7071067811865476-0.7071067811865476i, 0.7071067811865476+0.7071067811865476i, 0.7071067811865476-0.7071067811865476i, 0.7071067811865476+0.7071067811865476i, 0.7071067811865476-0.7071067811865476i, 0.7071067811865476-0.7071067811865476i, 0.7071067811865476+0.7071067811865476i, -0.7071067811865476+0.7071067811865476i, -0.7071067811865476+0.7071067811865476i, -0.7071067811865476+0.7071067811865476i, 0.7071067811865476-0.7071067811865476i, 0.7071067811865476-0.7071067811865476i, -0.7071067811865476+0.7071067811865476i, -0.7071067811865476-0.7071067811865476i, -0.7071067811865476-0.7071067811865476i, 0.7071067811865476-0.7071067811865476i, -0.7071067811865476-0.7071067811865476i, 0.7071067811865476+0.7071067811865476i, 0.7071067811865476-0.7071067811865476i, -0.7071067811865476+0.7071067811865476i, 0.7071067811865476+0.7071067811865476i, 0.7071067811865476-0.7071067811865476i, -0.7071067811865476-0.7071067811865476i, -0.7071067811865476+0.7071067811865476i, -0.7071067811865476-0.7071067811865476i, -0.7071067811865476-0.7071067811865476i, 0.7071067811865476-0.7071067811865476i, -0.7071067811865476+0.7071067811865476i, 0.7071067811865476+0.7071067811865476i, -0.7071067811865476-0.7071067811865476i, -0.7071067811865476+0.7071067811865476i, -0.7071067811865476+0.7071067811865476i, 0.7071067811865476+0.7071067811865476i, -0.7071067811865476-0.7071067811865476i, 0.7071067811865476+0.7071067811865476i, -0.7071067811865476-0.7071067811865476i, 0.7071067811865476+0.7071067811865476i, 0.7071067811865476+0.7071067811865476i, 0.7071067811865476+0.7071067811865476i, -0.7071067811865476+0.7071067811865476i, 0.7071067811865476-0.7071067811865476i, 0.7071067811865476+0.7071067811865476i, -0.7071067811865476-0.7071067811865476i, 0.7071067811865476+0.7071067811865476i, 0.7071067811865476-0.7071067811865476i, 0.7071067811865476-0.7071067811865476i, 0.7071067811865476+0.7071067811865476i, -0.7071067811865476-0.7071067811865476i, -0.7071067811865476+0.7071067811865476i, 0.7071067811865476+0.7071067811865476i, 0.7071067811865476-0.7071067811865476i, -0.7071067811865476-0.7071067811865476i, -0.7071067811865476-0.7071067811865476i, -0.7071067811865476-0.7071067811865476i, 0.7071067811865476-0.7071067811865476i, 0.7071067811865476-0.7071067811865476i, 0.7071067811865476+0.7071067811865476i, 0.7071067811865476-0.7071067811865476i, -0.7071067811865476-0.7071067811865476i, 0.7071067811865476+0.7071067811865476i, -0.7071067811865476+0.7071067811865476i, -0.7071067811865476-0.7071067811865476i, -0.7071067811865476+0.7071067811865476i, -0.7071067811865476+0.7071067811865476i, 0.7071067811865476-0.7071067811865476i, -0.7071067811865476+0.7071067811865476i, -0.7071067811865476+0.7071067811865476i, 0.7071067811865476-0.7071067811865476i, -0.7071067811865476+0.7071067811865476i, -0.7071067811865476-0.7071067811865476i, 0.7071067811865476-0.7071067811865476i, 0.7071067811865476+0.7071067811865476i, -0.7071067811865476-0.7071067811865476i, -0.7071067811865476-0.7071067811865476i, 0.7071067811865476-0.7071067811865476i, -0.7071067811865476-0.7071067811865476i, 0.7071067811865476-0.7071067811865476i, 0.7071067811865476-0.7071067811865476i, 0.7071067811865476+0.7071067811865476i, 0.7071067811865476+0.7071067811865476i, -0.7071067811865476-0.7071067811865476i, -0.7071067811865476+0.7071067811865476i, -0.7071067811865476+0.7071067811865476i, 0.7071067811865476-0.7071067811865476i, -0.7071067811865476-0.7071067811865476i, -0.7071067811865476+0.7071067811865476i, -0.7071067811865476-0.7071067811865476i, -0.7071067811865476+0.7071067811865476i, 0.7071067811865476-0.7071067811865476i, 0.7071067811865476+0.7071067811865476i, 0.7071067811865476+0.7071067811865476i, 0.7071067811865476-0.7071067811865476i, -0.7071067811865476-0.7071067811865476i, -0.7071067811865476+0.7071067811865476i, -0.7071067811865476+0.7071067811865476i, -0.7071067811865476-0.7071067811865476i, -0.7071067811865476-0.7071067811865476i, -0.7071067811865476+0.7071067811865476i, -0.7071067811865476+0.7071067811865476i, -0.7071067811865476+0.7071067811865476i, -0.7071067811865476+0.7071067811865476i, 0.7071067811865476+0.7071067811865476i, 0.7071067811865476+0.7071067811865476i, 0.7071067811865476+0.7071067811865476i, 0.7071067811865476-0.7071067811865476i, 0.7071067811865476-0.7071067811865476i, -0.7071067811865476+0.7071067811865476i, -0.7071067811865476+0.7071067811865476i, -0.7071067811865476+0.7071067811865476i, -0.7071067811865476-0.7071067811865476i, 0.7071067811865476-0.7071067811865476i, -0.7071067811865476+0.7071067811865476i, -0.7071067811865476+0.7071067811865476i, -0.7071067811865476-0.7071067811865476i, -0.7071067811865476+0.7071067811865476i, -0.7071067811865476-0.7071067811865476i, 0.7071067811865476+0.7071067811865476i, 0.7071067811865476+0.7071067811865476i, 0.7071067811865476+0.7071067811865476i, -0.7071067811865476-0.7071067811865476i, 0.7071067811865476-0.7071067811865476i, -0.7071067811865476+0.7071067811865476i, -0.7071067811865476-0.7071067811865476i, -0.7071067811865476+0.7071067811865476i, 0.7071067811865476+0.7071067811865476i, 0.7071067811865476-0.7071067811865476i, -0.7071067811865476+0.7071067811865476i, -0.7071067811865476-0.7071067811865476i, 0.7071067811865476-0.7071067811865476i, 0.7071067811865476-0.7071067811865476i, -0.7071067811865476-0.7071067811865476i, 0.7071067811865476-0.7071067811865476i, 0.7071067811865476-0.7071067811865476i, 0.7071067811865476-0.7071067811865476i, 0.7071067811865476+0.7071067811865476i, 0.7071067811865476-0.7071067811865476i, -0.7071067811865476+0.7071067811865476i, 0.7071067811865476+0.7071067811865476i, 0.7071067811865476+0.7071067811865476i, -0.7071067811865476-0.7071067811865476i, 0.7071067811865476+0.7071067811865476i, -0.7071067811865476-0.7071067811865476i, 0.7071067811865476-0.7071067811865476i, 0.7071067811865476+0.7071067811865476i, -0.7071067811865476+0.7071067811865476i, -0.7071067811865476+0.7071067811865476i, -0.7071067811865476-0.7071067811865476i, 0.7071067811865476-0.7071067811865476i, -0.7071067811865476-0.7071067811865476i, -0.7071067811865476+0.7071067811865476i, 0.7071067811865476-0.7071067811865476i, -0.7071067811865476+0.7071067811865476i, 0.7071067811865476-0.7071067811865476i, 0.7071067811865476-0.7071067811865476i, 0.7071067811865476+0.7071067811865476i, -0.7071067811865476+0.7071067811865476i, -0.7071067811865476-0.7071067811865476i, -0.7071067811865476+0.7071067811865476i, -0.7071067811865476-0.7071067811865476i, 0.7071067811865476-0.7071067811865476i, 0.7071067811865476+0.7071067811865476i, -0.7071067811865476+0.7071067811865476i, -0.7071067811865476-0.7071067811865476i, -0.7071067811865476-0.7071067811865476i, -0.7071067811865476-0.7071067811865476i, -0.7071067811865476-0.7071067811865476i, 0.7071067811865476+0.7071067811865476i, 0.7071067811865476+0.7071067811865476i, -0.7071067811865476+0.7071067811865476i, -0.7071067811865476-0.7071067811865476i, 0.7071067811865476-0.7071067811865476i, -0.7071067811865476-0.7071067811865476i, -0.7071067811865476-0.7071067811865476i, 0.7071067811865476-0.7071067811865476i, 0.7071067811865476+0.7071067811865476i, 0.7071067811865476-0.7071067811865476i, -0.7071067811865476-0.7071067811865476i, 0.7071067811865476-0.7071067811865476i, -0.7071067811865476+0.7071067811865476i, 0.7071067811865476-0.7071067811865476i, -0.7071067811865476+0.7071067811865476i, 0.7071067811865476+0.7071067811865476i, 0.7071067811865476+0.7071067811865476i, -0.7071067811865476+0.7071067811865476i, 0.7071067811865476+0.7071067811865476i, 0.7071067811865476-0.7071067811865476i, 0.7071067811865476-0.7071067811865476i, -0.7071067811865476+0.7071067811865476i, -0.7071067811865476-0.7071067811865476i, -0.7071067811865476+0.7071067811865476i, 0.7071067811865476-0.7071067811865476i, 0.7071067811865476-0.7071067811865476i, 0.7071067811865476+0.7071067811865476i, -0.7071067811865476-0.7071067811865476i, -0.7071067811865476-0.7071067811865476i, 0.7071067811865476+0.7071067811865476i, -0.7071067811865476-0.7071067811865476i, -0.7071067811865476-0.7071067811865476i, 0.7071067811865476-0.7071067811865476i, -0.7071067811865476+0.7071067811865476i, 0.7071067811865476-0.7071067811865476i, -0.7071067811865476-0.7071067811865476i, 0.7071067811865476+0.7071067811865476i, -0.7071067811865476+0.7071067811865476i, -0.7071067811865476+0.7071067811865476i, -0.7071067811865476+0.7071067811865476i, 0.7071067811865476+0.7071067811865476i, 0.7071067811865476-0.7071067811865476i, 0.7071067811865476+0.7071067811865476i, -0.7071067811865476-0.7071067811865476i, 0.7071067811865476-0.7071067811865476i, 0.7071067811865476+0.7071067811865476i, -0.7071067811865476-0.7071067811865476i, -0.7071067811865476+0.7071067811865476i, 0.7071067811865476-0.7071067811865476i, 0.7071067811865476-0.7071067811865476i, 0.7071067811865476-0.7071067811865476i, -0.7071067811865476-0.7071067811865476i, 0.7071067811865476-0.7071067811865476i, 0.7071067811865476+0.7071067811865476i, 0.7071067811865476-0.7071067811865476i, -0.7071067811865476+0.7071067811865476i, 0.7071067811865476-0.7071067811865476i, 0.7071067811865476+0.7071067811865476i, 0.7071067811865476-0.7071067811865476i, 0.7071067811865476+0.7071067811865476i, 0.7071067811865476-0.7071067811865476i, 0.7071067811865476+0.7071067811865476i, 0.7071067811865476+0.7071067811865476i, 0.7071067811865476+0.7071067811865476i, -0.7071067811865476+0.7071067811865476i, 0.7071067811865476+0.7071067811865476i, 0.7071067811865476+0.7071067811865476i, 0.7071067811865476-0.7071067811865476i, 0.7071067811865476+0.7071067811865476i, -0.7071067811865476-0.7071067811865476i, 0.7071067811865476+0.7071067811865476i, 0.7071067811865476+0.7071067811865476i, 0.7071067811865476-0.7071067811865476i, -0.7071067811865476+0.7071067811865476i, -0.7071067811865476-0.7071067811865476i, 0.7071067811865476+0.7071067811865476i, 0.7071067811865476-0.7071067811865476i, 0.7071067811865476-0.7071067811865476i, 0.7071067811865476-0.7071067811865476i, -0.7071067811865476-0.7071067811865476i, 0.7071067811865476+0.7071067811865476i, 0.7071067811865476+0.7071067811865476i, -0.7071067811865476-0.7071067811865476i, -0.7071067811865476+0.7071067811865476i, -0.7071067811865476-0.7071067811865476i, 0.7071067811865476-0.7071067811865476i, 0.7071067811865476-0.7071067811865476i, -0.7071067811865476+0.7071067811865476i, 0.7071067811865476-0.7071067811865476i, -0.7071067811865476-0.7071067811865476i, 0.7071067811865476-0.7071067811865476i, -0.7071067811865476+0.7071067811865476i, 0.7071067811865476+0.7071067811865476i, -0.7071067811865476+0.7071067811865476i, -0.7071067811865476+0.7071067811865476i, 0.7071067811865476+0.7071067811865476i, 0.7071067811865476+0.7071067811865476i, 0.7071067811865476-0.7071067811865476i, 0.7071067811865476-0.7071067811865476i, -0.7071067811865476-0.7071067811865476i, -0.7071067811865476+0.7071067811865476i, 0.7071067811865476+0.7071067811865476i, -0.7071067811865476-0.7071067811865476i, -0.7071067811865476-0.7071067811865476i, -0.7071067811865476-0.7071067811865476i, -0.7071067811865476+0.7071067811865476i, 0.7071067811865476-0.7071067811865476i, -0.7071067811865476+0.7071067811865476i, 0.7071067811865476+0.7071067811865476i, 0.7071067811865476-0.7071067811865476i, -0.7071067811865476+0.7071067811865476i, -0.7071067811865476+0.7071067811865476i, 0.7071067811865476-0.7071067811865476i]
  out "symbols":cdb[](array[numeric]) format="%.3f"
  out "output bit stream 2":i8[](array[numeric]) caption="output bit stream"
  out "output array":cdb[][](array[numeric])
  out "Total Size":i32
  out "appended array":i8[](array[numeric])
  out "Output Complex Data":cdb[](array[numeric])
  in  "Tab Control 3":enum32{"Parameters", "Debug", "CFO"}(tab)
  in  "Number of samples 2":i64=1600
  out "Coerced IQ rate 2":dbl=100000.0 format="%#_6p"
  in  "stop 3":bool
  out "Output bit stream 2":i8[](array[numeric]) caption="output bit stream"
  out "error out 4":errorcluster
  out "error out 5":errorcluster
  out "CFOest (Hz) 2":dbl[](array[numeric])
  out "Magnitude 2":dbl[](graph)
  out "Phase 2":dbl[](graph)
  out "FFT {X} 2":dbl[](graph)
  out "theta 2":dbl[](graph)
  out "Unequalized Data 2":cdb[](graph)
  out "Equalized Data 2":cdb[](graph)
  out "output bit stream 3":i8[][](array[numeric])
  # "Communication Parameters"
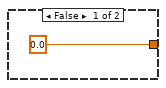
[diagram p3: hidden frame]
diagram:
  n1 = flat-sequence {
    tunnel: [w20] -> w15
    tunnel: w13 -> [w21]
    tunnel: [w19] -> w12
    tunnel: [w18] -> w11
    tunnel: [w17] -> w10
    tunnel: [w16] -> w3
    tunnel: w15 -> [w121]
    tunnel: [w120] -> w14
    tunnel: w12 -> [w119]
    tunnel: w11 -> [w118]
    tunnel: w10 -> [w117]
    tunnel: [w119] -> w8
    tunnel: [w118] -> w6
    tunnel: [w117] -> w4
    tunnel: w3 -> [w116]
    tunnel: [w116] -> w1
    tunnel: [w182] -> w9
    tunnel: w8 -> [w182]
    tunnel: [w181] -> w7
    tunnel: w6 -> [w181]
    tunnel: [w180] -> w5
    tunnel: w4 -> [w180]
    tunnel: [w179] -> w2
    tunnel: w1 -> [w179]
    tunnel: w9 -> [w191]
    tunnel: w7 -> [w190]
    tunnel: w5 -> [w189]
    tunnel: w2 -> [w188]
    frame #0 {
      n2 = case shown="0, Default" w21 {
        tunnel: [_ w26] -> w20
        tunnel: [_ "IQ rate"] -> w19
        tunnel: [_ "Carrier frequency"] -> w18
        tunnel: [_ "Gain"] -> w17
        tunnel: [_ "Device names"] -> w16
        frame 1 {
        }
        frame 0, Default {
          (unwired) TRUE ("number of samples is finite")
          # "1."
          n3 = call <instrlib>:"niUSRP Open Rx Session.vi"("device names"="Device names", "error in (no error)"=errorcluster {"status"=FALSE, "code"=0, "source"=""}) -> ("session handle out"=w28:refnum<k15>, "error out"=w27:errorcluster)  [unwired: 12 in]
          n4 = call <instrlib>:"niUSRP Configure Signal.vi"("session handle"=w28, "IQ rate"="IQ rate", "carrier frequency"="Carrier frequency", "gain"="Gain", "error in (no error)"=w27, "active antenna"="Active antenna") -> ("session handle out"=w30:refnum<k15>, "coerced IQ rate"=w31:dbl, "error out"=w29:errorcluster)  [unwired: 5 in, 2 out]
          "Coerced IQ rate" <- w31
          n5 = call <instrlib>:"niUSRP Initiate.vi"("session handle"=w30, "error in (no error)"=w29) -> ("session handle out"=w41:refnum<k15>, "error out"=w40:errorcluster)  [unwired: 12 in]
          n6 = while {
            tunnel: w41 -> [w85]
            tunnel: w40 -> [w80]
            tunnel: [w84] -> w34
            tunnel: "Number of samples" -> [w81]
            tunnel: w31 -> [w87]
            tunnel: [w86] -> w37
            tunnel: [w43] -> w26
            stop <- "stop" stop-if-true
            w69 = 8 ("dimension size")
            # "2."
            # "3."
            n7 = call-poly <instrlib>:"niUSRP Fetch Rx Data (poly).vi"("session handle"=w85, "number of samples"=w81, "error in (no error)"=w80) -> ("session handle out"=w84:refnum<k15>, "data"=w82:cdb[], "error out"=w83:errorcluster)  [unwired: 9 in, 1 out]
            "error out" <- w83
            n8 = call "VanDeBeek.vi"("Input"=w82) -> ("Phase"=→"Phase":dbl[], "Magnitude"=→"Magnitude":dbl[], "Indices"=w77:i32[], "CFOest (Hz)"=w76:dbl[])  [unwired: 6 in, 1 out]
            n9 = Divide(x=w87, y=256.0 ("x")) -> (x/y=w78:dbl)
            n10 = Multiply(x=w76, y=w78) -> (x*y=w73:dbl[])
            "CFOest (Hz)" <- w73
            n11 = for {
              tunnel: w73 -> [w107]
              workers-P: _ -> [_]
              tunnel: w87 -> [w106]
              tunnel: w83 -> [w105]
              tunnel: [w104] -> w86
              tunnel: w77 -> [w99] mode=indexing
              tunnel: w82 -> [w102]
              tunnel: [w96] -> w63 mode=indexing
              i -> [w97]
              w98 = 256  # N-Point FFT Size
              w101 = 64  # CP Size
              w109 = cdb[] [0.7071067811865476+0.7071067811865476i, 0.7071067811865476-0.7071067811865476i, -0.7071067811865476+0.7071067811865476i, -0.7071067811865476-0.7071067811865476i]  # 4QAM MAP
              w100 = 320  # Frame
              # "10."
              # "9."
              # "8."
              # "7."
              # "6."
              # "5."
              # "4."
              n12 = call "CP Removal.vi"("Input"=w102, "Indicies"=w99, "i"=w97, "Frame Size"=w100, "CP Size"=w101, "N-Point FFT Size"=w98) -> ("Output Without CP"=w103:cdb[])  [unwired: 9 in]
              n13 = call "CFO Correction.vi"("fs"=w106, "CFOest (freq)"=w107, "Index"=w97, "Input"=w103) -> ("Output"=w110:cdb[])  [unwired: 7 in]
              n14 = call-poly <vilib>:"FFT.vi"("FFT size"=256, "shift?"=TRUE, "X"=w110) -> ("FFT {X}"=w111:cdb[])  [unwired: 7 in, 1 out]
              n15 = Complex To Polar(r * e^(i*theta)=w111) -> (r=→"FFT {X}":dbl[], theta=→"theta":dbl[])
              n16 = call "Zero Pad Removal and Deinterleave.vi"("Input"=w111) -> ("Ref"=w95:cdb[], "Data"=w93:cdb[])  [unwired: 9 in]
              "Unequalized Data" <- w93
              n17 = call "Channel Estimation Linear.vi"("Ref"=w95) -> ("Hest"=w94:cdb[])  [unwired: 10 in]
              n18 = Multiply(x=w93, y=w94) -> (x*y=w108:cdb[])
              "Equalized Data" <- w108
              n19 = call-poly <vilib>:"MT Map Symbols to Bits.vi"("symbols"=w108, "symbol map"=w109, "error in (no error)"=w105) -> ("output bit stream"=w96:i8[], "error out"=w104:errorcluster)  [unwired: 11 in]
            }
            "output bit stream" <- w63
            n20 = String To Byte Array(string="Transmitter address\nreceiver address\ntime duration\nframe control\nframe check sequence") -> (unsigned byte array=w57:u8[])
            n21 = for {
              tunnel: w57 -> [w90] mode=indexing
              tunnel: [w88] -> w56 mode=indexing
              n22 = Number To Boolean Array(number=w90) -> (Boolean array=w89:bool[])
              n23 = Boolean To (0,1)(Boolean=w89) -> (0, 1=w88:i16[])
            }
            n24 = To Byte Integer(number=w56) -> (8bit integer=w53:i8[][])
            n25 = Array Size(array=w53) -> (size(s)=w55:i32[])
            n26 = Multiply Array Elements(1:w55) -> (0:w54:i32)
            n27 = Reshape Array(w53, w54) -> (w50:i8[])
            "output array 2" <- w50
            n28 = Delete From Array(array=w50, length=48, index=0) -> (deleted portion=w44:i8[])  [unwired: 1 out]
            n29 = Array Size(array=w63) -> (size(s)=w65:i32[])
            n30 = Multiply Array Elements(1:w65) -> (0:w66:i32)
            n31 = Reshape Array(w63, w66) -> (w61:i8[])
            "output array 3" <- w61
            n32 = Delete From Array(array=w61, length=48, index=0) -> (deleted portion=w42:i8[])  [unwired: 1 out]
            n33 = Subtract(x=w44, y=w42) -> (x-y=w48:i8[])
            n34 = Not Equal To 0?(x=w61) -> (x != 0?=w67:bool[])
            n35 = Array Size(array=w67) -> (size(s)=w68:i32)
            n36 = Absolute Value(x=w48) -> (abs(x)=w47:i8[])
            n37 = Quotient & Remainder(x=w68, y=w69) -> (floor(x/y)=w64:i32)  [unwired: 1 out]
            n38 = Add Array Elements(numeric array=w47) -> (sum=w45:i8)
            "sum" <- w45
            n39 = Reshape Array(w67, w64, w69) -> (w70:bool[][])
            n40 = Equal?(x=0.0, y=w45) -> (x = y?=w43:bool)
            "Reference Signal \n(RTS) Received" <- w43
            n41 = for {
              tunnel: w70 -> [w92] mode=indexing
              tunnel: [w91] -> w71 mode=indexing
              n42 = Boolean Array To Number(Boolean array=w92) -> (number=w91:u32)
            }
            n43 = To Unsigned Byte Integer(number=w71) -> (unsigned 8bit integer=w72:u8[])
            n44 = Byte Array To String(unsigned byte array=w72) -> (string=→"Received Message":string)
          }
          n45 = call <instrlib>:"niUSRP Abort.vi"("session handle"=w34, "error in (no error)"=w37) -> ("session handle out"=w35:refnum<k15>, "error out"=w36:errorcluster)  [unwired: 12 in]
          n46 = call <instrlib>:"niUSRP Close Session.vi"("session handle"=w35, "error in (no error)"=w36) -> ("error out"=→"error out 2":errorcluster)  [unwired: 13 in]
        }
      }
    }
    frame #1 {
      n47 = case shown="True" w121 {
        tunnel: [0.0 _] -> w120
        tunnel: w119 -> [_ w126]
        tunnel: w118 -> [_ w125]
        tunnel: w117 -> [_ w124]
        tunnel: w116 -> [_ w123]
        frame False {
        }
        frame True {
          w134 = cdb[] [0.7071067811865476+0.7071067811865476i, 0.7071067811865476-0.7071067811865476i, -0.7071067811865476+0.7071067811865476i, -0.7071067811865476-0.7071067811865476i]  # 4QAM MAP
          # "1."
          n48 = call <instrlib>:"niUSRP Open Tx Session.vi"("device names"=w123, "reset"=TRUE, "error in (no error)"="error in (no error)") -> ("session handle out"=w131:refnum<k15>, "error out"=w132:errorcluster)  [unwired: 11 in]
          n49 = Add(x=w126, y=w125) -> (x+y=w128:dbl)
          n50 = property class="niUSRP"(reference=w131, error in=w132, "LO Frequency"=w128) -> (reference out=w135:refnum<k15>, error out=w133:errorcluster)
          n51 = call <instrlib>:"niUSRP Configure Signal.vi"("session handle"=w135, "IQ rate"=w126, "carrier frequency"=w125, "gain"=w124, "error in (no error)"=w133, "active antenna"="TX1") -> ("session handle out"=w130:refnum<k15>, "coerced IQ rate"=→"coerced IQ rate":dbl)  [unwired: 5 in, 3 out]
          n52 = while {
            tunnel: w130 -> [w162]
            tunnel: [w161] -> w140
            tunnel: [w160] -> w139
            tunnel: w134 -> [w159]
            i -> [w142]
            stop <- w141 stop-if-true
            w158 = 125 ("y")
            # "10."
            # "8"
            # "3"
            # "2."
            # "1"
            n53 = Equal?(x=0.0, y=w142) -> (x = y?=w141:bool)
            "CTS is send" <- w141
            n54 = String To Byte Array(string="Now you can \ntransmit\nyour data, i am not \ngoing to interrupt \nyou  at all ") -> (unsigned byte array=w152:u8[])
            n55 = for {
              tunnel: w152 -> [w167] mode=indexing
              tunnel: [w165] -> w151 mode=indexing
              n56 = Number To Boolean Array(number=w167) -> (Boolean array=w166:bool[])
              n57 = Boolean To (0,1)(Boolean=w166) -> (0, 1=w165:i16[])
            }
            n58 = To Byte Integer(number=w151) -> (8bit integer=w148:i8[][])
            n59 = Array Size(array=w148) -> (size(s)=w150:i32[])
            n60 = Multiply Array Elements(1:w150) -> (0:w149:i32)
            n61 = Reshape Array(w148, w149) -> (w147:i8[])
            "output bit stream 2" <- w147
            "appended array" <- w147
            n62 = call-poly <vilib>:"MT Map Bits to Symbols.vi"("input bit stream"=w147, "symbol map"=w159) -> ("symbols"=w146:cdb[], "error out"=w157:errorcluster)  [unwired: 12 in]
            "Outgoing Constellation" <- w146
            "symbols" <- w146
            n63 = Array Size(array=w146) -> (size(s)=w164:i32)
            n64 = Divide(x=w164, y=w158) -> (x/y=w163:dbl)
            n65 = Reshape Array(w146, w163, w158) -> (w145:cdb[][])
            "output array" <- w145
            n66 = for {
              tunnel: w145 -> [w175] mode=indexing
              tunnel: [w169] -> w155 mode=concatenating
              w176 = cdb[] [-0.7071067811865475-0.7071067811865475i, -0.7071067811865475-0.7071067811865475i, -0.7071067811865475-0.7071067811865475i, 0.7071067811865475-0.7071067811865475i, 0.7071067811865475-0.7071067811865475i, 0.7071067811865475+0.7071067811865475i, 0.7071067811865475-0.7071067811865475i, -0.7071067811865475-0.7071067811865475i, 0.7071067811865475+0.7071067811865475i, -0.7071067811865475+0.7071067811865475i, -0.7071067811865475-0.7071067811865475i, -0.7071067811865475+0.7071067811865475i, -0.7071067811865475+0.7071067811865475i, 0.7071067811865475-0.7071067811865475i, -0.7071067811865475+0.7071067811865475i, -0.7071067811865475+0.7071067811865475i, 0.7071067811865475-0.7071067811865475i, -0.7071067811865475+0.7071067811865475i, -0.7071067811865475-0.7071067811865475i, 0.7071067811865475-0.7071067811865475i, 0.7071067811865475+0.7071067811865475i, -0.7071067811865475-0.7071067811865475i, -0.7071067811865475-0.7071067811865475i, 0.7071067811865475-0.7071067811865475i, -0.7071067811865475-0.7071067811865475i, 0.7071067811865475-0.7071067811865475i, 0.7071067811865475-0.7071067811865475i, 0.7071067811865475+0.7071067811865475i, 0.7071067811865475+0.7071067811865475i, -0.7071067811865475-0.7071067811865475i, -0.7071067811865475+0.7071067811865475i, -0.7071067811865475+0.7071067811865475i, 0.7071067811865475-0.7071067811865475i, -0.7071067811865475-0.7071067811865475i, -0.7071067811865475+0.7071067811865475i, -0.7071067811865475-0.7071067811865475i, -0.7071067811865475+0.7071067811865475i, 0.7071067811865475-0.7071067811865475i, 0.7071067811865475+0.7071067811865475i, 0.7071067811865475+0.7071067811865475i, 0.7071067811865475-0.7071067811865475i, -0.7071067811865475-0.7071067811865475i, -0.7071067811865475+0.7071067811865475i, -0.7071067811865475+0.7071067811865475i, -0.7071067811865475-0.7071067811865475i, -0.7071067811865475-0.7071067811865475i, -0.7071067811865475+0.7071067811865475i, -0.7071067811865475+0.7071067811865475i, -0.7071067811865475+0.7071067811865475i, -0.7071067811865475+0.7071067811865475i]  # Reference Symbols
              # "7"
              # "6"
              # "5"
              # "4"
              n67 = Array Size(array=w175) -> (size(s)=→"Data Size":i32)
              n68 = call "Data Reference Interleave.vi"("Data Symbols"=w175, "Reference Symbols"=w176) -> ("Interleaved Output"=w173:cdb[])  [unwired: 9 in]
              "Interleaved Output" <- w173
              n69 = Array Size(array=w173) -> (size(s)=→"Reference Symbols \n         Added":i32)
              n70 = call "Zero Padding.vi"("Array in"=w173) -> ("Array out"=w171:cdb[])  [unwired: 10 in]
              "Array out" <- w171
              n71 = Array Size(array=w171) -> (size(s)=→"After Zero \n  Padding":i32)
              n72 = call-poly <vilib>:"Inverse FFT.vi"("shift?"=TRUE, "FFT {X}"=w171) -> ("X"=w177:cdb[])  [unwired: 8 in, 1 out]
              "X" <- w177
              n73 = call "CP Insertion.vi"("Input"=w177) -> ("Output with CP"=w169:cdb[])  [unwired: 10 in]
              "Output with CP" <- w169
              n74 = Array Size(array=w169) -> (size(s)=→"After CP":i32)
            }
            n75 = Multiply(x=w155, y=0.5 ("value")) -> (x*y=w154:cdb[])
            "Output Complex Data" <- w154
            n76 = Array Size(array=w154) -> (size(s)=→"Total Size":i32)
            n77 = call-poly <instrlib>:"niUSRP Write Tx Data (poly).vi"("session handle"=w162, "data"=w154, "error in (no error)"=w157) -> ("session handle out"=w160:refnum<k15>, "error out"=w161:errorcluster)  [unwired: 11 in]
          }
          n78 = call <instrlib>:"niUSRP Close Session.vi"("session handle"=w139, "error in (no error)"=w140) -> ("error out"=→"error out 3":errorcluster)  [unwired: 13 in]
        }
      }
    }
    frame #2 {
      n79 = while {
        i -> [w185]
        stop <- w184 stop-if-true
        n80 = Wait Until Next ms Multiple(millisecond multiple=u32 5000) -> (millisecond timer value=→"millisecond timer to \n    Receive Signal":u32)
        n81 = Equal?(x=0.0, y=w185) -> (x = y?=w184:bool)
      }
    }
    frame #3 {
      (unwired) TRUE ("number of samples is finite")
      # "1."
      n82 = call <instrlib>:"niUSRP Open Rx Session.vi"("device names"=w188, "error in (no error)"=errorcluster {"status"=FALSE, "code"=0, "source"=""}) -> ("session handle out"=w194:refnum<k15>, "error out"=w193:errorcluster)  [unwired: 12 in]
      n83 = call <instrlib>:"niUSRP Configure Signal.vi"("session handle"=w194, "IQ rate"=w191, "carrier frequency"=w190, "gain"=w189, "error in (no error)"=w193, "active antenna"="RX1") -> ("session handle out"=w196:refnum<k15>, "coerced IQ rate"=w197:dbl, "error out"=w195:errorcluster)  [unwired: 5 in, 2 out]
      "Coerced IQ rate 2" <- w197
      n84 = call <instrlib>:"niUSRP Initiate.vi"("session handle"=w196, "error in (no error)"=w195) -> ("session handle out"=w206:refnum<k15>, "error out"=w205:errorcluster)  [unwired: 12 in]
      n85 = while {
        tunnel: w206 -> [w225]
        tunnel: w205 -> [w220]
        tunnel: [w224] -> w200
        tunnel: "Number of samples 2" -> [w221]
        tunnel: w197 -> [w227]
        tunnel: [w226] -> w203
        stop <- "stop 3" stop-if-true
        # "2."
        # "3."
        n86 = call-poly <instrlib>:"niUSRP Fetch Rx Data (poly).vi"("session handle"=w225, "number of samples"=w221, "error in (no error)"=w220) -> ("session handle out"=w224:refnum<k15>, "data"=w222:cdb[], "error out"=w223:errorcluster)  [unwired: 9 in, 1 out]
        "error out 4" <- w223
        n87 = call "VanDeBeek.vi"("Input"=w222) -> ("Phase"=→"Phase 2":dbl[], "Magnitude"=→"Magnitude 2":dbl[], "Indices"=w217:i32[], "CFOest (Hz)"=w216:dbl[])  [unwired: 6 in, 1 out]
        n88 = Divide(x=w227, y=256.0 ("x")) -> (x/y=w218:dbl)
        n89 = Multiply(x=w216, y=w218) -> (x*y=w213:dbl[])
        "CFOest (Hz) 2" <- w213
        n90 = for {
          tunnel: w213 -> [w243]
          workers-P: _ -> [_]
          tunnel: w227 -> [w242]
          tunnel: w223 -> [w241]
          tunnel: [w240] -> w226
          tunnel: w217 -> [w235] mode=indexing
          tunnel: w222 -> [w238]
          tunnel: [w232] -> w210 mode=indexing
          i -> [w233]
          w234 = 256  # N-Point FFT Size
          w237 = 64  # CP Size
          w245 = cdb[] [0.7071067811865476+0.7071067811865476i, 0.7071067811865476-0.7071067811865476i, -0.7071067811865476+0.7071067811865476i, -0.7071067811865476-0.7071067811865476i]  # 4QAM MAP
          w236 = 320  # Frame
          # "10."
          # "9."
          # "8."
          # "7."
          # "6."
          # "5."
          # "4."
          n91 = call "CP Removal.vi"("Input"=w238, "Indicies"=w235, "i"=w233, "Frame Size"=w236, "CP Size"=w237, "N-Point FFT Size"=w234) -> ("Output Without CP"=w239:cdb[])  [unwired: 9 in]
          n92 = call "CFO Correction.vi"("fs"=w242, "CFOest (freq)"=w243, "Index"=w233, "Input"=w239) -> ("Output"=w246:cdb[])  [unwired: 7 in]
          n93 = call-poly <vilib>:"FFT.vi"("FFT size"=256, "shift?"=TRUE, "X"=w246) -> ("FFT {X}"=w247:cdb[])  [unwired: 7 in, 1 out]
          n94 = Complex To Polar(r * e^(i*theta)=w247) -> (r=→"FFT {X} 2":dbl[], theta=→"theta 2":dbl[])
          n95 = call "Zero Pad Removal and Deinterleave.vi"("Input"=w247) -> ("Ref"=w231:cdb[], "Data"=w229:cdb[])  [unwired: 9 in]
          "Unequalized Data 2" <- w229
          n96 = call "Channel Estimation Linear.vi"("Ref"=w231) -> ("Hest"=w230:cdb[])  [unwired: 10 in]
          n97 = Multiply(x=w229, y=w230) -> (x*y=w244:cdb[])
          "Equalized Data 2" <- w244
          n98 = call-poly <vilib>:"MT Map Symbols to Bits.vi"("symbols"=w244, "symbol map"=w245, "error in (no error)"=w241) -> ("output bit stream"=w232:i8[], "error out"=w240:errorcluster)  [unwired: 11 in]
          "Output bit stream 2" <- w232
        }
        "output bit stream 3" <- w210
        n99 = Array Size(array=w210) -> (size(s)=w211:i32[])
        n100 = Multiply Array Elements(1:w211) -> (0:w212:i32)
        n101 = Reshape Array(w210, w212) -> (w209:i8[])
        n102 = call-poly <vilib>:"Binary to Digital.vi"("binary array"=w209) -> ("digital waveform"=w208:digitalwaveform)  [unwired: 9 in, 1 out]
        n103 = call-poly <vilib>:"Digital to Analog.vi"("digital waveform"=w208) -> ("analog waveform"=→"analog waveform" →"Received Signal":waveform(dbl))  [unwired: 7 in, 3 out]
      }
      n104 = call <instrlib>:"niUSRP Abort.vi"("session handle"=w200, "error in (no error)"=w203) -> ("session handle out"=w201:refnum<k15>, "error out"=w202:errorcluster)  [unwired: 12 in]
      n105 = call <instrlib>:"niUSRP Close Session.vi"("session handle"=w201, "error in (no error)"=w202) -> ("error out"=→"error out 5":errorcluster)  [unwired: 13 in]
    }
  }
  n106 = feedback-in #1(w14) -> ()
  n107 = feedback #1() -> (w13:dbl)  [unwired: 1 in]
